vi "conv_FreQ_Pos.vi"(6 "data_in":dbl[][](array[numeric]), 8 "error in":errorcluster, 11 "Freq":dbl=30.0) -> (0 "error out":errorcluster, 3 "Pos":dbl, 4 "data_out":dbl[][](array[numeric]))   [LabVIEW 2019]
uses:
  <vilib>/Utility/file.llb/Read Delimited Spreadsheet (DBL).vi
  <vilib>/gmath/NI_Gmath.lvlib
panel:
  out "array_Freq":dbl[](array[numeric])
  out "array_Pos":dbl[](array[numeric])
  out "yi":dbl[](array[numeric]) format="%_6g"
  out "xi used":dbl[](array[numeric]) format="%_6g"
  # "VI to convert vapor pressure of He4 or He3 to temperature.\n\ndata_out can/should be fed back to data_in \nso as to read the data file only once."
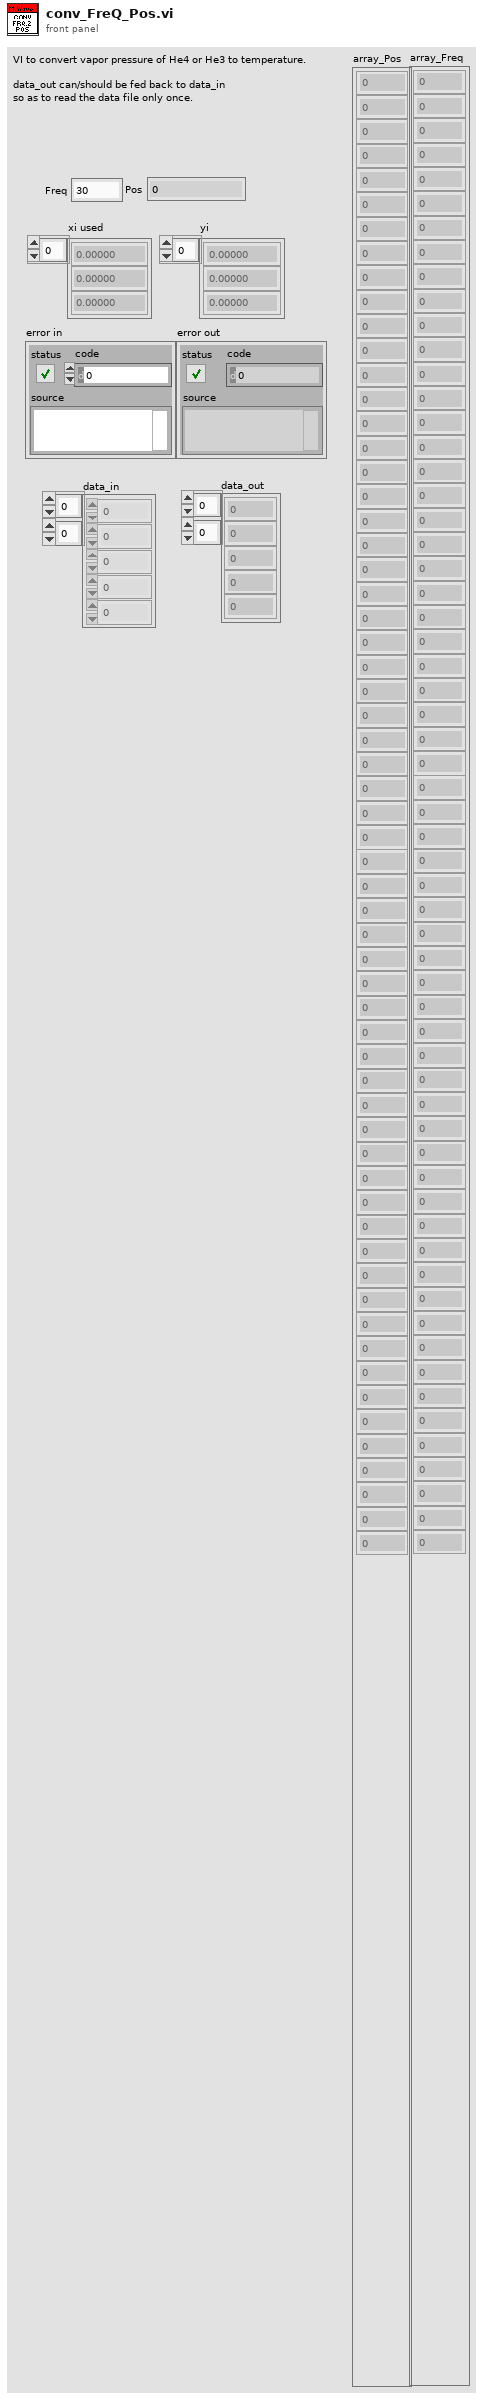
[diagram p1: front panel]
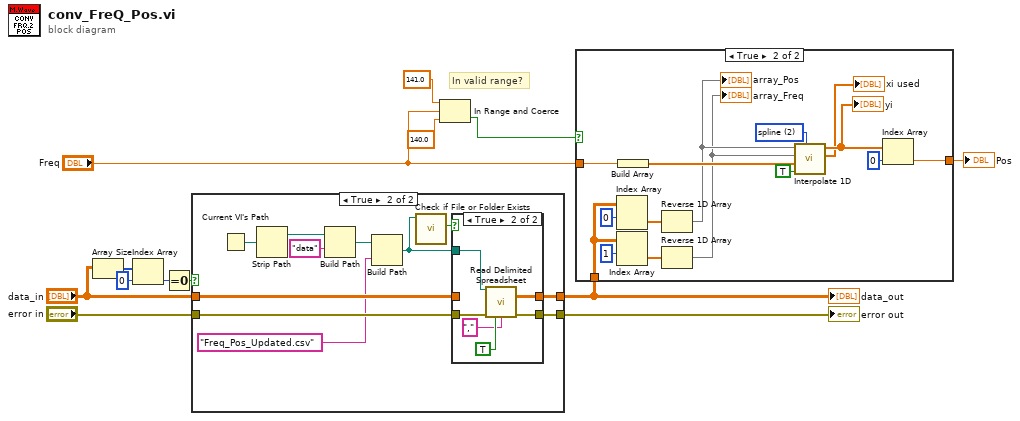
[diagram p0: block diagram]
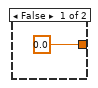
[diagram p2: hidden frame]
diagram:
  # "In valid range?"
  n1 = Array Size(array="data_in") -> (size(s)=w7:i32[])
  n2 = Index Array(array=w7, index=0) -> (element=w6:i32)
  n3 = Equal To 0?(x=w6) -> (x = 0?=w10:bool)
  n4 = case shown="True" w10 {
    tunnel: "error in" -> [w14 w20]
    tunnel: [w14 w19] -> w12
    tunnel: [w15 w18] -> w9
    tunnel: "data_in" -> [w15 w17]
    frame False {
    }
    frame True {
      n5 = Current VI's Path() -> (path=w26:path)
      n6 = Strip Path(path=w26) -> (stripped path=w25:path)  [unwired: 1 out]
      n7 = Build Path(base path=w25, name or relative path="data") -> (appended path=w23:path)
      n8 = Build Path(base path=w23, name or relative path="Freq_Pos_Updated.csv") -> (appended path=w21:path)
      n9 = call <vilib>:"Check if File or Folder Exists.vi"("path"=w21) -> ("file or folder exists?"=w22:bool)  [unwired: 8 in, 2 out]
      n10 = case shown="True" w22 {
        tunnel: w21 -> [_ w34]
        tunnel: w20 -> [w27 w33]
        tunnel: [w27 w32] -> w19
        tunnel: [w28 w31] -> w18
        tunnel: w17 -> [w28 _]
        frame False {
        }
        frame True {
          n11 = call-poly <vilib>:"Read Delimited Spreadsheet.vi"("file path (dialog if empty)"=w34, "error in (no error)"=w33, "transpose? (F)"=TRUE, "delimiter (\\t)"="," ("delimiter (\\t)")) -> ("all rows"=w31:dbl[][], "error out"=w32:errorcluster)  [unwired: 6 in, 4 out]
        }
      }
    }
  }
  "error out" <- w12
  "data_out" <- w9
  n12 = In Range and Coerce(upper limit=141.0, x="Freq", lower limit=140.0) -> (In Range?=w1:bool)  [unwired: 1 out]
  n13 = case shown="True" w1 {
    tunnel: w9 -> [_ w49]
    tunnel: [0.0 ("Numeric") w45] -> w8
    tunnel: "Freq" -> [_ w38]
    frame False {
    }
    frame True {
      w39 = 2 items=["nearest", "linear", "spline", "cubic Hermite", "Lagrange"] ("method")
      n14 = Index Array(array=w49, index (row)=0) -> (element=w42:dbl[])  [unwired: 1 in]
      n15 = Index Array(array=w49, index (row)=1) -> (element=w41:dbl[])  [unwired: 1 in]
      n16 = Build Array(w38) -> (w44:dbl[])
      n17 = Reverse 1D Array(array=w42) -> (reversed array=w37:dbl[])
      "array_Pos" <- w37
      n18 = Reverse 1D Array(array=w41) -> (reversed array=w36:dbl[])
      "array_Freq" <- w36
      n19 = call <vilib>:"Interpolate 1D.vi"("method"=w39, "X is monotonic"=TRUE, "xi"=w44, "X"=w36, "Y"=w37) -> ("xi used"=→"xi used":dbl[], "yi"=w47:dbl[])  [unwired: 4 in, 1 out]
      "yi" <- w47
      n20 = Index Array(array=w47, index=0) -> (element=w45:dbl)
    }
  }
  "Pos" <- w8
